vi "tsapp_enable_bus_statistics.vi"(8 "error in (no error)":errorcluster caption="错误输入（无错误）", 10 "AEnable":bool, 11 "路径输入":path) -> (0 "error out":errorcluster caption="错误输出", 2 "retuen":i32, 3 "路径输出":path)   [LabVIEW 2014]
doc: "Function Introduction:\nEnable bus statistics timer to calculate bus statistics\nCall location :\ninput parameter :\nAEnable: Enable bus statistics timer\nReturn value :\n==0: Execution successful\nOther values: Query error code"
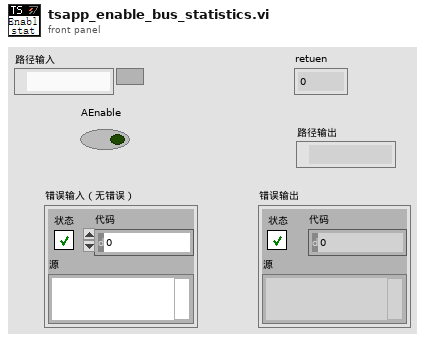
[diagram p1: front panel]
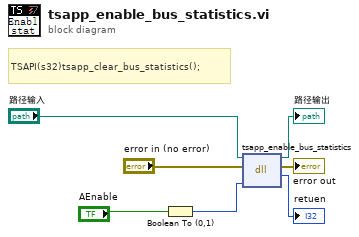
[diagram p0: block diagram]
diagram:
  # "TSAPI(s32)tsapp_clear_bus_statistics();"
  n1 = Boolean To (0,1)(Boolean="AEnable") -> (0, 1=w2:i16)
  n2 = dll-call lib="D:/Work/LabVIEW Code/TSMaster Labview SDK/LabVIEW/LabVIEW-TSMasterAPI_CLN/TSMasterAPI_LabVIEW-2024-08-02 09-14-06/Not_organized_vi/TSMaster.*" fn="tsapp_enable_bus_statistics"(path in="路径输入", error in="error in (no error)", "AEnable"=w2) -> (path out=→"路径输出":path, error out=→"error out":errorcluster, "返回类型"=→"retuen":u8)  [unwired: 2 in]
